vi "Named Service TCP Client.vi"() -> ()   [LabVIEW 2014]
doc: "This VI implements a client for the named service created by Named Service TCP Server.vi.\nThe client connects to the service using the name of the service and the address of the server. It receives the response from the server, displays it and closes the connection.\n\n<b>Note:</b> This VI is built to work with the Named Service TCP Server.vi in TCP.llb."
panel:
  out "?":string
  out "error out":errorcluster
  in  "error in":errorcluster
  # "Instructions:\n1. Open Named Service TCP Server.vi located in the same library.\n2. Follow the instructions on it's front panel.\n\nNote: This VI is built to work with the Named Service \nTCP Server.vi in TCP.llb."
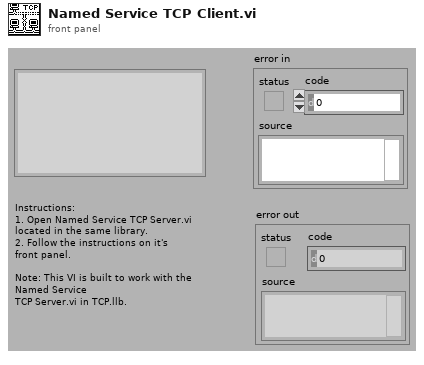
[diagram p1: front panel]
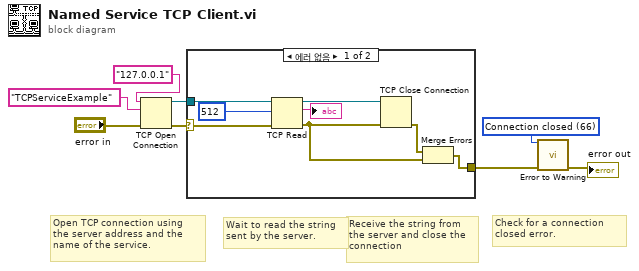
[diagram p0: block diagram]
diagram:
  w1 = 66 items=["No Error", "Argument Error", "Memory Full", "Out of Zone", "End of File", "File Already Open", "Generic File IO Error", "File Not Found", "File Permission Error", "Disk Full", "Duplicate Path", "Too Many Files Open", "Not Enabled", "Resource File Not Found", "Cannot Add Resource", "Resource Not Found", "Image Not Found", "Image Memory Error", "Pen Does Not Exist", "Config Bad Type", "Config Token Not Found", "Config Parse Error", "Config Memory Error", "Bad External Code Format", "Bad External Code Offset", "External Code Not Present", "Null Window", "Destroy Window Mixup", "Null Menu", "Print Aborted", "Bad Print Record", "Print Driver Error", "Windows Error During Print", "Memory Error During Print", "Print Dialog Error", "Generic Print Error", "Invalid Device Refnum", "Device Not Found", "Device Parameter Error", "Device Unit Error", "Can't Open Device", "Device Call Aborted", "Generic Error", "Cancelled By User", "Object ID Too Low", "Object ID Too High", "Object Not In Heap", "Unknown Heap", "Bad DefProc ID", "DefProc Not In Table", "Message Out Of Range", "Null Method", "Unknown Message", "Manager Call Not Supported", "Bad address", "Connection In progress", "Connection timed out", "Connection is already in progress", "Network attribute not supported", "Network error", "Address in use", "System out of memory", "Connection aborted", "Connection refused", "Connection is not connected", "Connection is already connected", "Connection closed", "Initialize error (interapplication manager)", "Bad occurrence", "Wait on unbound occurrence handler", "Occurrence queue overflow", "Bad path", "Semaphore not signaled", "Unrecognized type (interapplication manager)"] ("1st Error to Convert")
  # "Wait to read the string\nsent by the server."
  # "Check for a connection \nclosed error."
  # "Receive the string from\nthe server and close the\nconnection"
  # "Open TCP connection using\nthe server address and the\nname of the service."
  n1 = TCP Open Connection(address="127.0.0.1", remote port or service name="TCPServiceExample", error in (no error)="error in") -> (connection ID=w6:refnum<k5>, error out=w7:errorcluster)  [unwired: 2 out]
  n2 = case shown="에러 없음" w7 {
    selector: w7 -> [w11 w17]
    tunnel: [w12 w17] -> w3
    tunnel: w6 -> [w16 _]
    frame No Error {
      n3 = TCP Read(connection ID=w16, bytes to read=512, error in (no error)=w11) -> (connection ID out=w10:refnum<k5>, data out=→"?":string, error out=w9:errorcluster)  [unwired: 2 out]
      n4 = TCP Close Connection(connection ID=w10, error in (no error)=w9) -> (error out=w13:errorcluster)  [unwired: 2 out]
      n5 = Merge Errors(w13, w9) -> (w12:errorcluster)
    }
    frame Error {
    }
  }
  n6 = call <vilib>:"Error to Warning.vi"("1st Error to Convert"=w1, "error in"=w3) -> ("warning out"=→"error out":errorcluster)  [unwired: 4 in, 9 out]
